vi "Write TCPComEvents.vi"(8 "error in (no error)":errorcluster, 10 "TCPComEvents.lvclass":refnum<class "TCPComEvents.lvclass">, 11 "TCPCommunicator in":refnum<class "TCPCommunicator.lvclass">) -> (0 "error out":errorcluster, 3 "TCPCommunicator out":refnum<class "TCPCommunicator.lvclass">)   [LabVIEW 2016, in "TCPCommunicator.lvclass"]
uses:
  TCPCommunicator.lvclass
  TCPComEvents/TCPComEvents.lvclass
  TCPCommunicator.lvclass/TCPCommunicator.ctl
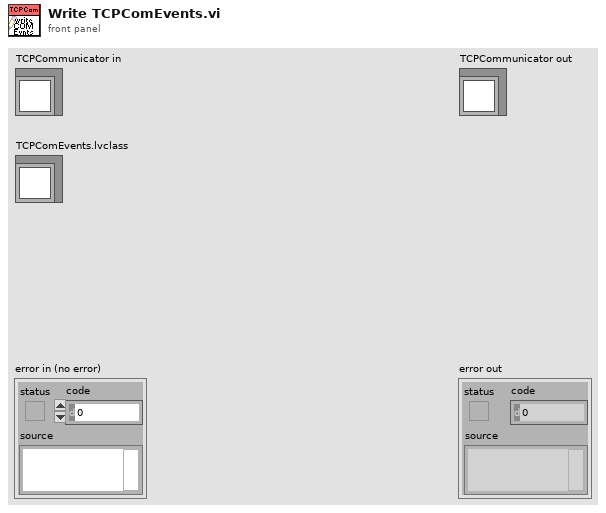
[diagram p1: front panel]
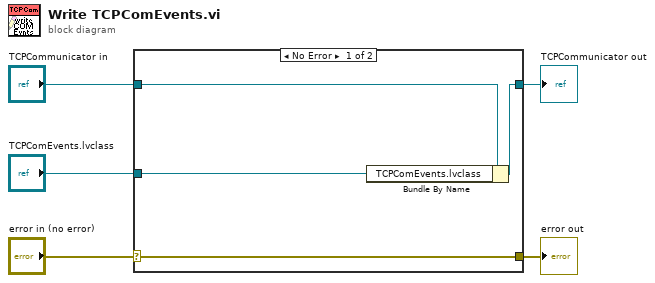
[diagram p0: block diagram]
diagram:
  n1 = case shown="No Error" "error in (no error)" {
    selector: "error in (no error)" -> [w9 w10]
    tunnel: [w9 w10] -> w4
    tunnel: [w7 w11] -> w2
    tunnel: "TCPCommunicator in" -> [w8 w11]
    tunnel: "TCPComEvents.lvclass" -> [w6 _]
    frame No Error {
      n2 = Bundle By Name(cluster=w8, "TCPComEvents.lvclass"=w6) -> (w7:refnum<class "TCPCommunicator.lvclass">)
    }
    frame Error {
    }
  }
  "error out" <- w4
  "TCPCommunicator out" <- w2
